vi "Equalize Denumerator.vi"(10 "High Res Arithmetic in":refnum<class "Rational Number.lvclass">, 11 "Rational Number In":refnum<class "Rational Number.lvclass">) -> (2 "High Res Arithmetic 3":refnum<class "Rational Number.lvclass">, 3 "Rational Number Out":refnum<class "Rational Number.lvclass">)   [LabVIEW 2021, in "Rational Number.lvclass"]
uses:
  Rational Number.lvclass
  Rational Number.lvclass/Rational Number.ctl
  <vilib>/gmath/NI_AAL_MathFunc.lvlib
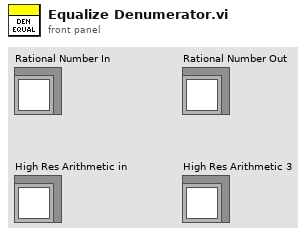
[diagram p1: front panel]
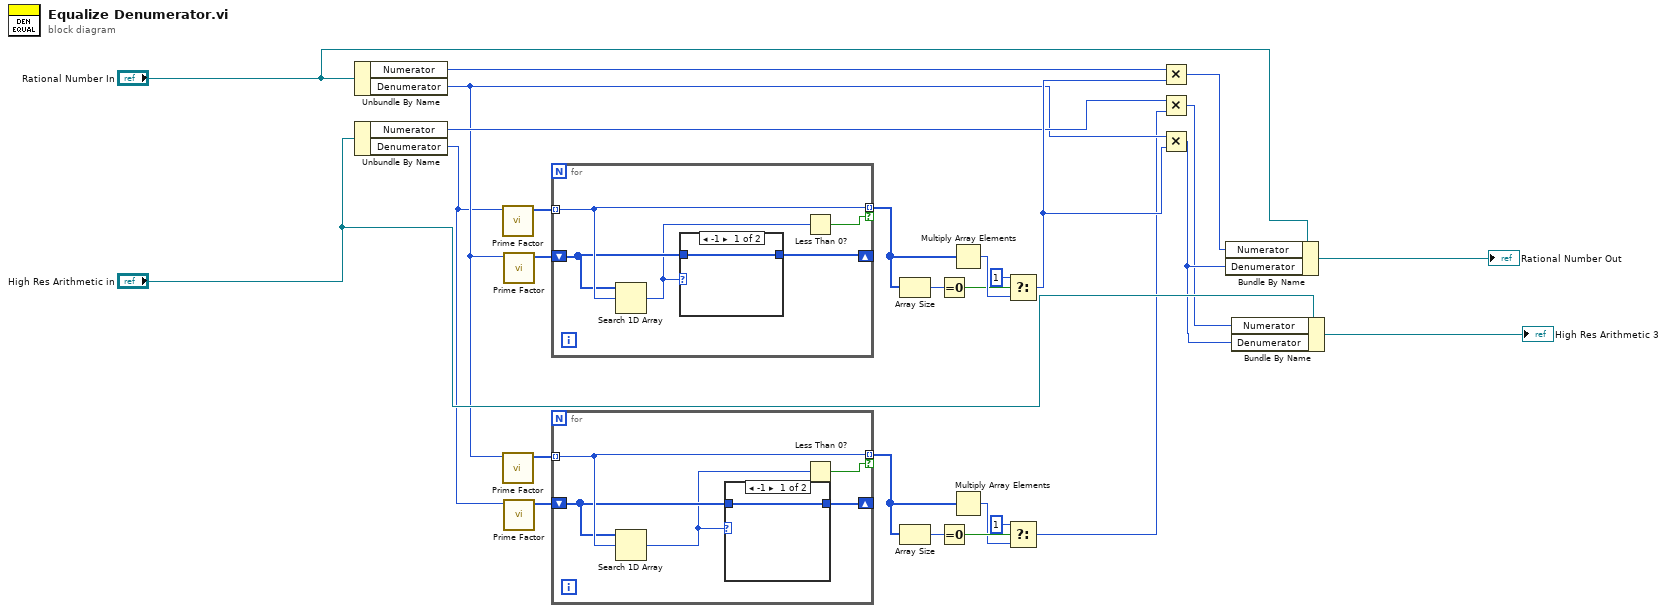
[diagram p0: block diagram]
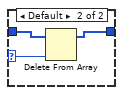
[diagram p2: hidden frame]
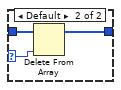
[diagram p3: hidden frame]
diagram:
  n1 = Unbundle By Name("Rational Number In") -> ("Numerator"=w14:i64, "Denumerator"=w3:i64)
  n2 = Unbundle By Name("High Res Arithmetic in") -> ("Numerator"=w13:i64, "Denumerator"=w2:i64)
  n3 = call <vilib>:"Prime Factor.vi"("n"=w2) -> ("Prime Factors"=w15:i64[])  [unwired: 9 in]
  n4 = call <vilib>:"Prime Factor.vi"("n"=w3) -> ("Prime Factors"=w8:i64[])  [unwired: 9 in]
  n5 = call <vilib>:"Prime Factor.vi"("n"=w3) -> ("Prime Factors"=w11:i64[])  [unwired: 9 in]
  n6 = call <vilib>:"Prime Factor.vi"("n"=w2) -> ("Prime Factors"=w10:i64[])  [unwired: 9 in]
  n7 = for {
    tunnel: w15 -> [w32] mode=indexing
    tunnel: [w32] -> w12 mode=indexing if=w31
    shift-right: [w29] -> _
    shift-left: w11 -> [w30]
    n8 = Search 1D Array(1D array=w30, element=w32) -> (index of element=w28:i32)  [unwired: 1 in]
    n9 = case shown="-1" w28 {
      selector: w28 -> [_ w34]
      tunnel: w30 -> [w33 w36]
      tunnel: [w33 w35] -> w29
      frame -1 {
      }
      frame Default {
        n10 = Delete From Array(array=w36, index=w34) -> (array with subset deleted=w35:i64[])  [unwired: 1 in, 1 out]
      }
    }
    n11 = Less Than 0?(x=w28) -> (x < 0?=w31:bool)
  }
  n12 = for {
    tunnel: w8 -> [w41] mode=indexing
    tunnel: [w41] -> w9 mode=indexing if=w40
    shift-right: [w38] -> _
    shift-left: w10 -> [w39]
    n13 = Search 1D Array(1D array=w39, element=w41) -> (index of element=w37:i32)  [unwired: 1 in]
    n14 = case shown="-1" w37 {
      selector: w37 -> [_ w43]
      tunnel: w39 -> [w42 w45]
      tunnel: [w42 w44] -> w38
      frame -1 {
      }
      frame Default {
        n15 = Delete From Array(array=w45, index=w43) -> (array with subset deleted=w44:i64[])  [unwired: 1 in, 1 out]
      }
    }
    n16 = Less Than 0?(x=w37) -> (x < 0?=w40:bool)
  }
  n17 = Array Size(array=w12) -> (size(s)=w16:i32)
  n18 = Array Size(array=w9) -> (size(s)=w7:i32)
  n19 = Equal To 0?(x=w16) -> (x = 0?=w17:bool)
  n20 = Equal To 0?(x=w7) -> (x = 0?=w6:bool)
  n21 = Multiply Array Elements(1:w12) -> (0:w18:i64)
  n22 = Multiply Array Elements(1:w9) -> (0:w5:i64)
  n23 = Select(t=i64 1, s=w17, f=w18) -> (s? t:f=w20:i64)
  n24 = Select(t=i64 1, s=w6, f=w5) -> (s? t:f=w1:i64)
  n25 = Multiply(x=w14, y=w20) -> (x*y=w21:i64)
  n26 = Multiply(x=w13, y=w1) -> (x*y=w22:i64)
  n27 = Multiply(x=w3, y=w20) -> (x*y=w23:i64)
  n28 = Bundle By Name(cluster="Rational Number In", "Numerator"=w21, "Denumerator"=w23) -> (→"Rational Number Out":refnum<class "Rational Number.lvclass">)
  n29 = Bundle By Name(cluster="High Res Arithmetic in", "Numerator"=w22, "Denumerator"=w23) -> (→"High Res Arithmetic 3":refnum<class "Rational Number.lvclass">)
